vi "Vector joystck.vi"(0 "Jx input":dbl=1.0 min=-1.0 max=1.0 format="%.4f", 1 "apply\nFILTER":bool, 2 "Reset\nFILTER":bool, 5 "Jy input":dbl=0.04 min=-1.0 max=1.0 format="%.4f", 7 "Jr input":dbl=1.0 min=-1.0 max=1.0 format="%.4f", 11 "error in (no error)":errorcluster) -> (4 "output cluster":T1 {"Jr" format="%.4g"; "theta (rad)" format="%_4f"; "R" format="%.4g"; "Jy" format="%.4g"; "theta (deg)" format="%_4f"; "Jx" format="%.4g"}, 15 "error out":errorcluster)   [LabVIEW 2023]
uses:
  ctrl defs/ctrl driver input.ctl
  <vilib>/Analysis/coordinate.llb/Angle Units.ctl
  <vilib>/Analysis/coordinate.llb/Angle Range (Degree).ctl
  <vilib>/Analysis/coordinate.llb/Wrap Angle (scalar).vi
  <vilib>/Analysis/NI_AAL_Angle.lvlib
panel:
  out "XY after\nDEADBAND":cluster{"X":dbl, "Y":dbl}={"X"=1.0, "Y"=0.04}
  out "Jr":dbl=1.0 format="%#.4f"
  in  "resting steer angle (deg)":dbl=90.0 format="%#_13g"
  in  "axis dead band":dbl=0.05000000000000004 format="%#_13g"
  in  "Max dx/dt":dbl=10.0
  out "Jy":dbl format="%#.4f"
  out "Jx":dbl=0.9992009587217894 format="%#.4f"
  out "Joystick":cluster{dbl[], dbl[]}(graph)={[0.0, 1.0], [0.0, 0.04]}
  out "theta (deg)":dbl=2.29061004263853
  out "theta (rad)":dbl=0.039978687123290044
  out "R":dbl=1.0
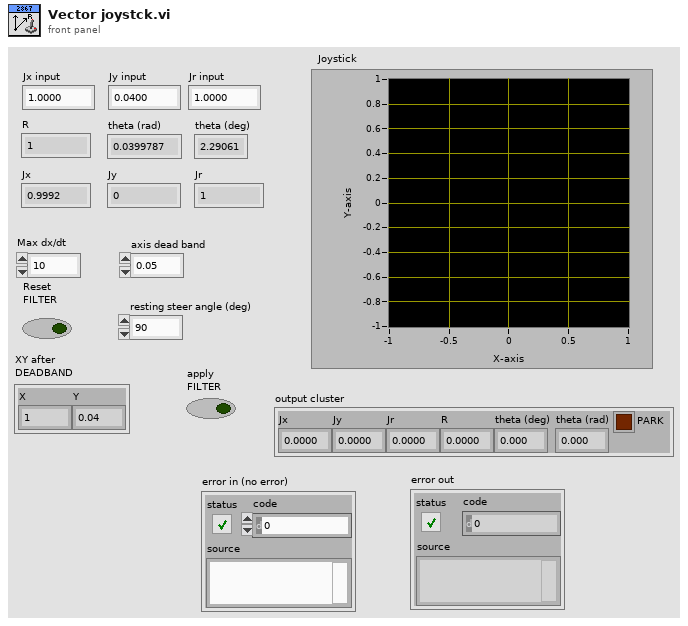
[diagram p1: front panel]
types:
  T1 = typedef "ctrl driver input.ctl" = cluster{"Jx":dbl, "Jy":dbl, "Jr ":dbl, "R":dbl, "theta (deg)":dbl, "theta (rad)":dbl, "PARK":bool}
  T2 = typedef "NI_AAL_Angle.lvlib/Angle Range (Degree).ctl" = u16
  T3 = typedef "NI_AAL_Angle.lvlib/Angle Units.ctl" = i32
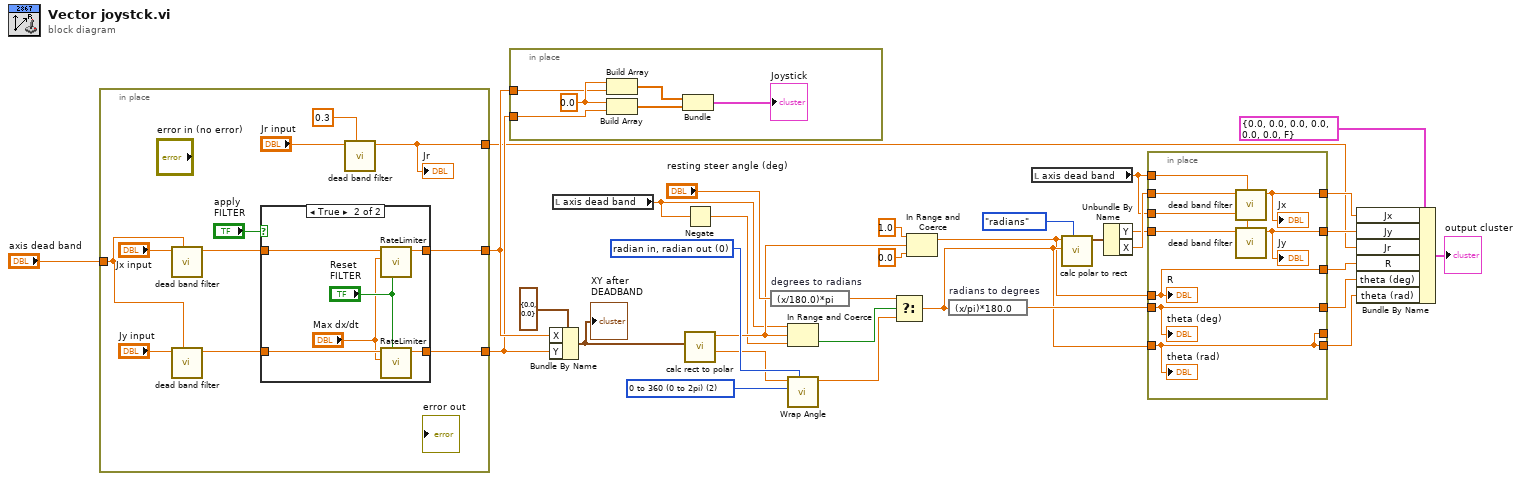
[diagram p0: block diagram]
diagram:
  w21 = T2 2 items=["none", "-180 to 180 (-pi to pi)", "0 to 360 (0 to 2pi)"] ("angle range")
  w22 = T3 0 items=["radian in, radian out", "radian in, degree out", "degree in, degree out", "degree in, radian out"] ("angle units")
  n1 = in-place {
    in-place-border: [w41] -> w28
    in-place-border: [w40] -> w27
    in-place-border: "axis dead band" -> [w38]
    in-place-border: [w34] -> w2
    n2 = call "dead band filter.vi"("deadband"=w38, "input"="Jx input") -> ("output"=w42:dbl)  [unwired: 9 in]
    n3 = call "dead band filter.vi"("deadband"=w38, "input"="Jy input") -> ("output"=w39:dbl)  [unwired: 9 in]
    n4 = case shown="True" "apply\nFILTER" {
      tunnel: w42 -> [w45 w52]
      tunnel: [w45 w51] -> w41
      tunnel: [w46 w50] -> w40
      tunnel: w39 -> [w46 w49]
      frame False {
      }
      frame True {
        n5 = call "RateLimiter.vi"("Reset"="Reset\nFILTER", "Max dx/dt"="Max dx/dt", "Input"=w52) -> ("Output"=w51:dbl)  [unwired: 8 in]
        n6 = call "RateLimiter.vi"("Reset"="Reset\nFILTER", "Max dx/dt"="Max dx/dt", "Input"=w49) -> ("Output"=w50:dbl)  [unwired: 8 in]
      }
    }
    n7 = call "dead band filter.vi"("deadband"=0.3, "input"="Jr input") -> ("output"=w34:dbl)  [unwired: 9 in]
    "Jr" <- w34
  }
  n8 = in-place {
    in-place-border: w28 -> [w57]
    in-place-border: w27 -> [w56]
    w58 = 0.0 ("element")
    n9 = Build Array(w58, w57) -> (w54:dbl[])
    n10 = Build Array(w58, w56) -> (w53:dbl[])
    n11 = Bundle(w54, w53) -> (→"Joystick":cluster{dbl[], dbl[]})  [unwired: 1 in]
  }
  n12 = Bundle By Name(cluster=cluster{"X":dbl, "Y":dbl} {"X"=0.0, "Y"=0.0} ("XY"), "X"=w28, "Y"=w27) -> (w15:cluster{"X":dbl, "Y":dbl})
  "XY after\nDEADBAND" <- w15
  n13 = local read "axis dead band"() -> (w11:dbl)
  n14 = Negate(x=w11) -> (-x=w10:dbl)
  n15 = call "calc rect to polar.vi"("XY"=w15) -> ("angle (rad)"=w17:dbl, "Magnitude"=w18:dbl)  [unwired: 8 in, 1 out]
  n16 = expression code="(x/180.0)*pi" "degrees to radians"("resting steer angle (deg)") -> (w12:dbl)
  n17 = In Range and Coerce(upper limit=w11, x=w18, lower limit=w10) -> (In Range?=w19:bool)  [unwired: 1 out]
  n18 = call-poly <vilib>:"Wrap Angle.vi"("angle units"=w22, "angle range"=w21, "angle in"=w17) -> ("angle out"=w14:dbl)  [unwired: 7 in, 1 out]
  n19 = Select(t=w12, s=w19, f=w14) -> (s? t:f=w30:dbl)
  n20 = In Range and Coerce(upper limit=1.0, x=w18, lower limit=0.0 ("x")) -> (coerced(x)=w29:dbl)  [unwired: 1 out]
  n21 = expression code="(x/pi)*180.0" "radians to degrees"(w30) -> (w31:dbl)
  n22 = local read "axis dead band"() -> (w9:dbl)
  n23 = call "calc polar to rect.vi"("units"=enum16{"degrees", "radians"}."radians", "angle"=w30, "mag"=w29) -> ("XY"=w23:cluster{"X":dbl, "Y":dbl})  [unwired: 8 in]
  n24 = Unbundle By Name(w23) -> ("Y"=w32:dbl, "X"=w33:dbl)
  n25 = in-place {
    in-place-border: w33 -> [w67]
    in-place-border: w32 -> [w66]
    in-place-border: w31 -> [w59]
    in-place-border: w30 -> [w60]
    in-place-border: w29 -> [w61]
    in-place-border: [w60] -> _
    in-place-border: w9 -> [w65]
    in-place-border: w9 -> [w64]
    in-place-border: [w63] -> w7
    in-place-border: [w62] -> w6
    in-place-border: [w61] -> w5
    in-place-border: [w60] -> w4
    in-place-border: [w59] -> w3
    n26 = call "dead band filter.vi"("deadband"=w64, "input"=w67) -> ("output"=w63:dbl)  [unwired: 9 in]
    "Jx" <- w63
    n27 = call "dead band filter.vi"("deadband"=w65, "input"=w66) -> ("output"=w62:dbl)  [unwired: 9 in]
    "Jy" <- w62
    "theta (deg)" <- w59
    "theta (rad)" <- w60
    "R" <- w61
  }
  n28 = Bundle By Name(cluster=T1 {"Jx"=0.0, "Jy"=0.0, "Jr "=0.0, "R"=0.0, "theta (deg)"=0.0, "theta (rad)"=0.0, "PARK"=FALSE} ("DRIVER INPUT"), "Jx"=w7, "Jy"=w6, "Jr"=w2, "R"=w5, "theta (deg)"=w3, "theta (rad)"=w4) -> (→"output cluster":T1)
